vi "Create Execution Profiler Result View.vi"(8 "error in (no error)":errorcluster, 11 "Execution Profiler Result View in":T1) -> (0 "error out":errorcluster, 3 "Execution Profiler Result View out":refnum<class "Execution Profiler Result View.lvclass">)   [LabVIEW 2020, in "Execution Profiler Result View.lvclass"]
uses:
  Execution Profiler Result View.lvclass
  Execution Profiler/Execution Profiler View Data.ctl
  Helper Classes/Open Test Case Interface/Open Test Case.lvclass
  Execution Profiler Result View.lvclass/Execution Profiler Result View.ctl
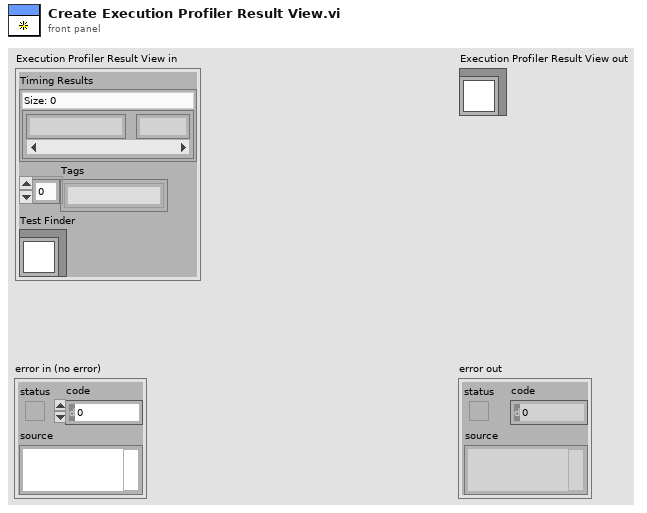
[diagram p1: front panel]
types:
  T1 = typedef "Execution Profiler Result View.lvclass/Execution Profiler View Data.ctl" = cluster{"Timing Results":map{string, dbl}, "Tags":string[], "Test Finder":refnum<class "Open Test Case.lvclass">}
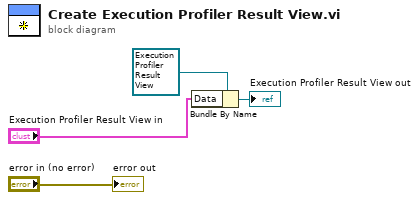
[diagram p0: block diagram]
diagram:
  n1 = Bundle By Name(cluster=refnum<class "Execution Profiler Result View.lvclass"> refnum ("Execution Profiler Result View out"), "Data"="Execution Profiler Result View in") -> (→"Execution Profiler Result View out":refnum<class "Execution Profiler Result View.lvclass">)
  "error out" <- "error in (no error)"
